vi "SubSystems.vi"(8 "error in":errorcluster) -> ()   [LabVIEW 2023]
doc: "This VI calls the various robot subsystems that will then run in parallel. New subSystems will automatlically script code to make the call."
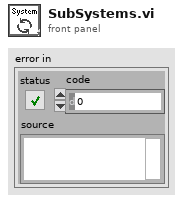
[diagram p1: front panel]
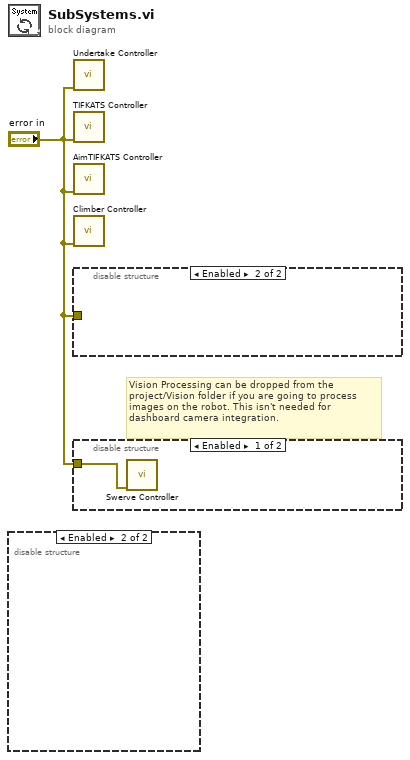
[diagram p0: block diagram]
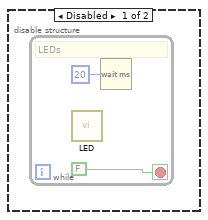
[diagram p3: hidden frame]
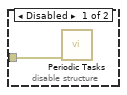
[diagram p4: hidden frame]
diagram:
  # "Vision Processing can be dropped from the\nproject/Vision folder if you are going to process\nimages on the robot. This isn't needed for\ndashboard camera integration."
  n1 = disable-structure shown="Enabled" {
    frame Disabled {
      n2 = while {
        stop <- FALSE stop-if-true
        # "LEDs"
        n3 = call "LED.vi"() -> ()  [unwired: 12 in]
        n4 = Wait (ms)(milliseconds to wait=u32 20) -> ()  [unwired: 1 out]
      }
    }
    frame Enabled {
    }
  }
  n5 = call "Undertake Controller.vi"("error in"="error in") -> ()  [unwired: 11 in]
  n6 = call "TIFKATS Controller.vi"("error in"="error in") -> ()  [unwired: 11 in]
  n7 = call "AimTIFKATS Controller.vi"("error in"="error in") -> ()  [unwired: 11 in]
  n8 = call "Climber Controller.vi"("error in"="error in") -> ()  [unwired: 11 in]
  n9 = disable-structure shown="Enabled" {
    disable-tunnel: "error in" -> [w4 _]
    frame Disabled {
      n10 = call "Periodic Tasks.vi"("error in"=w4) -> ()  [unwired: 1 in, 10 out]
    }
    frame Enabled {
    }
  }
  n11 = disable-structure shown="Enabled" {
    disable-tunnel: "error in" -> [w5 _]
    frame Enabled {
      n12 = call "Swerve Controller.vi"("error in"=w5) -> ()  [unwired: 11 in]
    }
    frame Disabled {
    }
  }
